vi "Clear Output.vi"(0 "PainOutputTerminal in":refnum<class "PainOutputTerminal.lvclass">, 11 "error in (no error)":errorcluster) -> (4 "PainOutputTerminal out":refnum<class "PainOutputTerminal.lvclass">, 15 "error out":errorcluster)   [LabVIEW 2016, in "PainOutputTerminal.lvclass"]
uses:
  PainOutputTerminal.lvclass
  PainOutputTerminal.lvclass/PainOutputTerminal.ctl
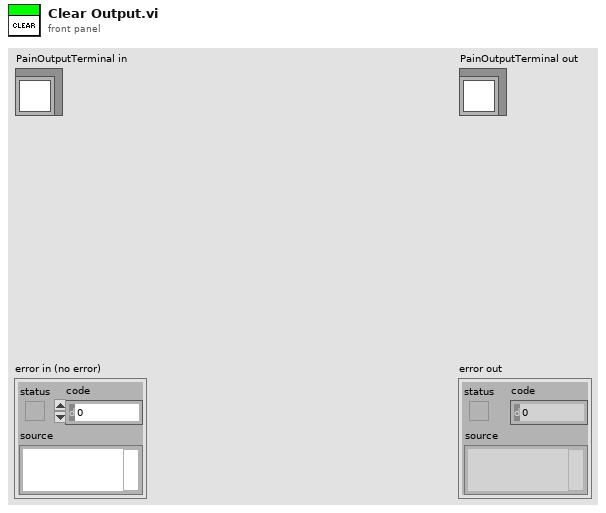
[diagram p1: front panel]
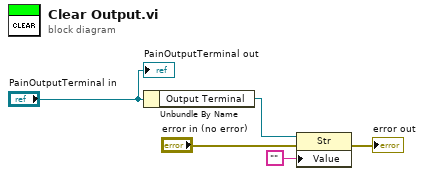
[diagram p0: block diagram]
diagram:
  n1 = Unbundle By Name("PainOutputTerminal in") -> ("Output Terminal"=w4:refnum<vi>)
  n2 = property class="Str"(reference=w4, error in="error in (no error)", "Value"="") -> (error out=→"error out":errorcluster)  [unwired: 1 out]
  "PainOutputTerminal out" <- "PainOutputTerminal in"
